vi "libssh2_knownhost_readfile - valid file - returns number of hosts.vi"() -> ()   [LabVIEW 2013, in "libssh2_tests.lvlib"]
uses:
  libssh2_tests.lvlib
  libssh2/libssh2_init_default.vi
  <vilib>/addons/_JKI Toolkits/Caraya/classes/Assert/Assert Equal Value_Variant.vi
  <vilib>/addons/_JKI Toolkits/Caraya/classes/Test/Test.lvclass
  libssh2/libssh2.lvlib
  <vilib>/addons/_JKI Toolkits/Caraya/classes/Assert/Assert.lvclass
panel:
  out "error out":errorcluster
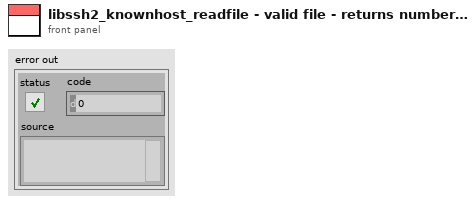
[diagram p1: front panel]
types:
  T1 = typedef "libssh2.lvlib/Session Refnum.ctl" = refnum<k1>
  T2 = typedef "libssh2.lvlib/Known Hosts Collection Refnum.ctl" = refnum<k1>
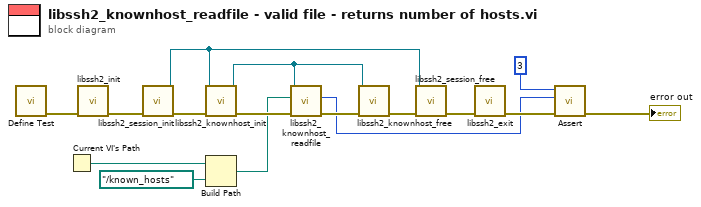
[diagram p0: block diagram]
diagram:
  n1 = call <vilib>:"Define Test.vi"() -> ("error out"=w15:errorcluster)  [unwired: 10 in, 1 out]
  n2 = Current VI's Path() -> (path=w3:path)
  n3 = call-poly "libssh2_init.vi"("error in (no error)"=w15) -> ("error out"=w14:errorcluster)  [unwired: 10 in]
  n4 = call "libssh2_session_init.vi"("error in (no error)"=w14) -> ("error out"=w13:errorcluster, "session"=w10:T1)  [unwired: 9 in]
  n5 = call "libssh2_knownhost_init.vi"("error in (no error)"=w13, "session"=w10) -> ("error out"=w8:errorcluster, "known hosts collection"=w6:T2)  [unwired: 8 in]
  n6 = Build Path(base path=w3, name or relative path=path "../known_hosts" ("filename")) -> (appended path=w1:path)
  n7 = call "libssh2_knownhost_readfile.vi"("error in (no error)"=w8, "filename"=w1, "known hosts collection"=w6) -> ("error out"=w7:errorcluster, "hosts added"=w5:i32)  [unwired: 7 in]
  n8 = call "libssh2_knownhost_free.vi"("error in (no error)"=w7, "known hosts collection"=w6) -> ("error out"=w9:errorcluster)  [unwired: 9 in]
  n9 = call "libssh2_session_free.vi"("error in (no error)"=w9, "session"=w10) -> ("error out"=w12:errorcluster)  [unwired: 9 in]
  n10 = call "libssh2_exit.vi"("error in (no error)"=w12) -> ("error out"=w11:errorcluster)  [unwired: 10 in]
  n11 = call-poly <vilib>:"Assert.vi"("error in (no error)"=w11, "Y"=w5, "X"=3 ("hosts added")) -> ("error out"=→"error out":errorcluster)  [unwired: 7 in, 1 out]
